vi "Hoaram.vi"(8 "lambda":T1, 9 "d":T2, 10 "T":dbl[](array[numeric])) -> (2 "F":dbl[](array[numeric]))   [LabVIEW 2013]
panel:
  in  "alphakont":dbl
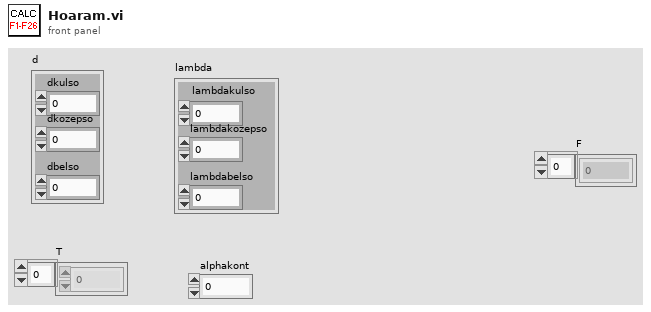
[diagram p1: front panel]
types:
  T1 = cluster{"lambdakulso":dbl, "lambdakozepso":dbl, "lambdabelso":dbl}
  T2 = cluster{"dkulso":dbl, "dkozepso":dbl, "dbelso":dbl}
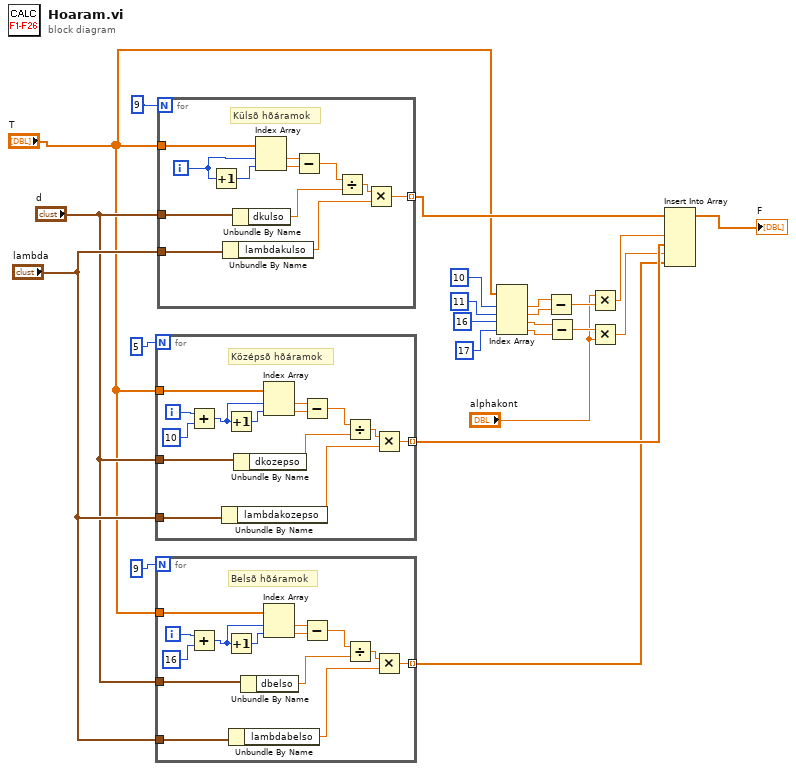
[diagram p0: block diagram]
diagram:
  n1 = for {
    N: 5 -> [_]
    tunnel: "T" -> [w36]
    tunnel: "d" -> [w31]
    tunnel: "lambda" -> [w30]
    tunnel: [w27] -> w3 mode=indexing
    i -> [w26]
    # "Középsõ hõáramok"
    n2 = Add(x=w26, y=10) -> (x+y=w25:i32)
    n3 = Unbundle By Name(w30) -> ("lambdakozepso"=w28:dbl)
    n4 = Increment(x=w25) -> (x+1=w37:i32)
    n5 = Unbundle By Name(w31) -> ("dkozepso"=w29:dbl)
    n6 = Index Array(array=w36, index #1=w25, index #2=w37) -> (element #1=w35:dbl, element #2=w34:dbl)
    n7 = Subtract(x=w35, y=w34) -> (x-y=w33:dbl)
    n8 = Divide(x=w33, y=w29) -> (x/y=w32:dbl)
    n9 = Multiply(x=w32, y=w28) -> (x*y=w27:dbl)
  }
  n10 = for {
    N: 9 -> [_]
    tunnel: "T" -> [w50]
    tunnel: "d" -> [w45]
    tunnel: "lambda" -> [w44]
    tunnel: [w41] -> w1 mode=indexing
    i -> [w40]
    # "Belsõ hõáramok"
    n11 = Add(x=w40, y=16) -> (x+y=w39:i32)
    n12 = Increment(x=w39) -> (x+1=w51:i32)
    n13 = Unbundle By Name(w44) -> ("lambdabelso"=w42:dbl)
    n14 = Unbundle By Name(w45) -> ("dbelso"=w43:dbl)
    n15 = Index Array(array=w50, index #1=w39, index #2=w51) -> (element #1=w49:dbl, element #2=w48:dbl)
    n16 = Subtract(x=w49, y=w48) -> (x-y=w47:dbl)
    n17 = Divide(x=w47, y=w43) -> (x/y=w46:dbl)
    n18 = Multiply(x=w46, y=w42) -> (x*y=w41:dbl)
  }
  n19 = for {
    N: 9 -> [_]
    tunnel: "T" -> [w61]
    tunnel: "d" -> [w56]
    tunnel: "lambda" -> [w55]
    tunnel: [w52] -> w18 mode=indexing
    i -> [w63]
    # "Külsõ hõáramok"
    n20 = Increment(x=w63) -> (x+1=w62:i32)
    n21 = Unbundle By Name(w55) -> ("lambdakulso"=w53:dbl)
    n22 = Unbundle By Name(w56) -> ("dkulso"=w54:dbl)
    n23 = Index Array(array=w61, index #1=w63, index #2=w62) -> (element #1=w60:dbl, element #2=w59:dbl)
    n24 = Subtract(x=w60, y=w59) -> (x-y=w58:dbl)
    n25 = Divide(x=w58, y=w54) -> (x/y=w57:dbl)
    n26 = Multiply(x=w57, y=w53) -> (x*y=w52:dbl)
  }
  n27 = Index Array(array="T", index #1=10 ("index"), index #2=11 ("index"), index #3=16 ("index"), index #4=17 ("index")) -> (element #1=w11:dbl, element #2=w10:dbl, element #3=w9:dbl, element #4=w8:dbl)
  n28 = Subtract(x=w11, y=w10) -> (x-y=w6:dbl)
  n29 = Subtract(x=w9, y=w8) -> (x-y=w7:dbl)
  n30 = Multiply(x="alphakont", y=w6) -> (x*y=w4:dbl)
  n31 = Multiply(x=w7, y="alphakont") -> (x*y=w2:dbl)
  n32 = Insert Into Array(array=w18, new element #1=w4, new element #2=w3, new element #3=w2, new element #4=w1) -> (→"F":dbl[])  [unwired: 1 in]
